vi "LWXPS_PositionerCompensatedFastPCOPrepare.vi"(0 "XPS Reference IN":refnum<k24>, 1 "Positioner Name":string, 2 "Scan Direction":i32, 3 "Start Position IN":dbl[](array[numeric]), 4 "Number of Items":i32, 5 "LabVIEW error IN":errorcluster) -> (14 "XPS Reference OUT":refnum<k24>, 15 "Returned error code":i32, 16 "Start Position OUT":dbl[](array[numeric]), 17 "XPS Error String":string, 19 "LabVIEW error OUT":errorcluster)   [LabVIEW 2014]
uses:
  D:/XPSQ8_LabView_Library/Development/Source/Dll/Newport.XPS.CommandInterface.dll
  Dll/Newport.XPS.CommandInterface.dll
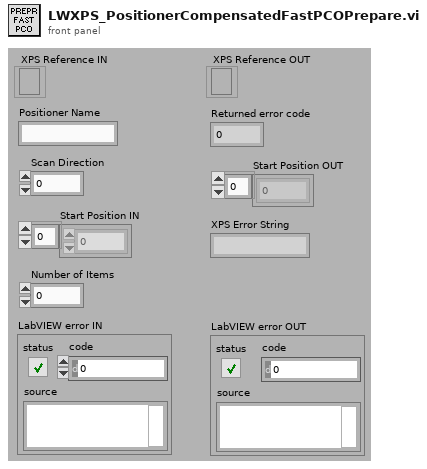
[diagram p1: front panel]
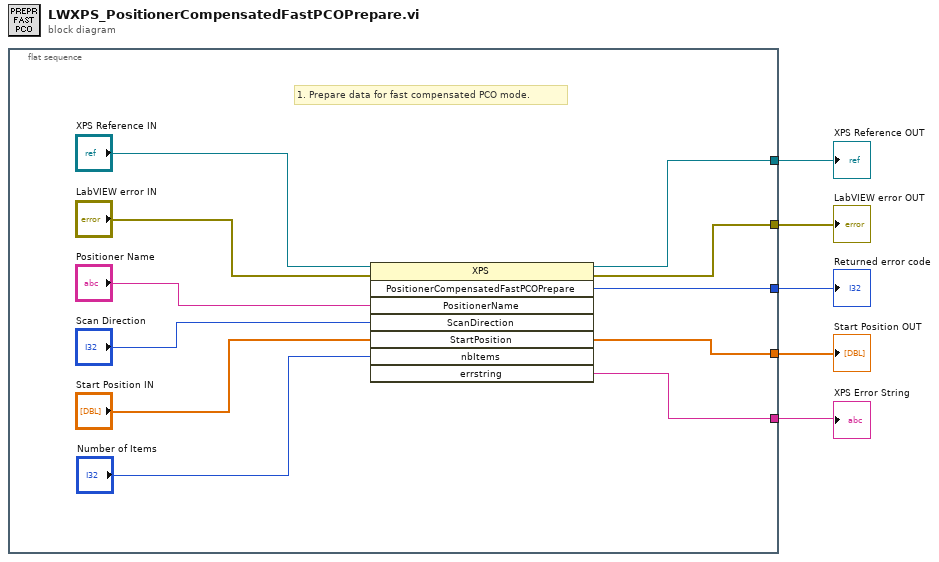
[diagram p0: block diagram]
diagram:
  n1 = flat-sequence {
    tunnel: [w11] -> w5
    tunnel: [w6] -> w4
    tunnel: [w13] -> w3
    tunnel: [w12] -> w2
    tunnel: [w10] -> w1
    frame #0 {
      # "1. Prepare data for fast compensated PCO mode."
      n2 = invoke class="XPS" method="PositionerCompensatedFastPCOPrepare"(reference="XPS Reference IN", error in="LabVIEW error IN", "PositionerName"="Positioner Name", "ScanDirection"="Scan Direction", "StartPosition"="Start Position IN", "nbItems"="Number of Items") -> (reference out=w11:refnum<k24>, error out=w6:errorcluster, "PositionerCompensatedFastPCOPrepare"=w13:i32, "StartPosition"=w12:dbl[], "errstring"=w10:string)  [unwired: 2 in, 3 out]
    }
  }
  "XPS Error String" <- w1
  "XPS Reference OUT" <- w5
  "LabVIEW error OUT" <- w4
  "Returned error code" <- w3
  "Start Position OUT" <- w2
